vi "błędy szerokość.vi"(4 "błąd szerokość":errorcluster) -> (1 "Błędy  szerokości":string)   [LabVIEW 2015, in "Biblioteka moduł map v3.lvlib" / "Konwersja wsp.lvlib" / "Obsługa błędów.lvlib"]
doc: "SubVI ma za zadanie sprawdzić czy wystąpiły błędy związane z szerokością. Jeżli tak to ma dopisać tekst informujący o błędach związanych z szerokością geograficzną."
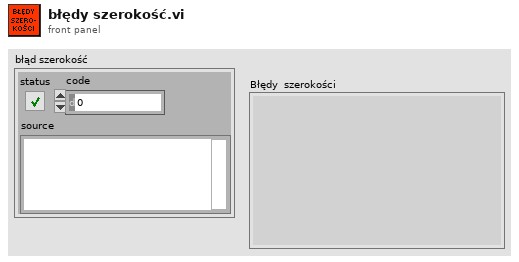
[diagram p1: front panel]
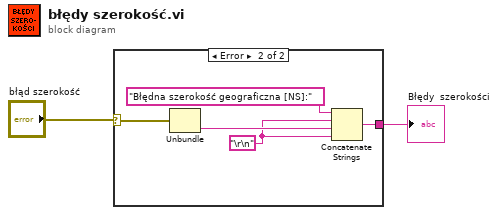
[diagram p0: block diagram]
diagram:
  n1 = case shown="Error" "błąd szerokość" {
    selector: "błąd szerokość" -> [_ w6]
    tunnel: [_ w3] -> w1
    frame No Error {
    }
    frame Error {
      w4 = "\r\n"
      n2 = Unbundle(w6) -> ("source"=w5:string)  [unwired: 2 out]
      n3 = Concatenate Strings("Błędna szerokość geograficzna [NS]:" ("source"), w4, w5, w4) -> (w3:string)
    }
  }
  "Błędy  szerokości" <- w1
